vi "update_modifier_values.vi"(0 "TrajectoryDL091126GenericVoxel in":refnum<class "TrajectoryDL091126GenericVoxel.lvclass">, 1 "position-dependently?":bool, 5 "x coordinates in":dbl[unit][](array[numeric]), 7 "y coordinates in":dbl[unit][](array[numeric]), 9 "z coordinates in":dbl[unit][](array[numeric]), 11 "error in (no error)":errorcluster) -> (4 "TrajectoryDL091126GenericVoxel out":refnum<class "TrajectoryDL091126GenericVoxel.lvclass">, 6 "x coordinates out":dbl[unit][](array[numeric]), 8 "y coordindates out":dbl[unit][](array[numeric]), 10 "z coordinates out":dbl[unit][](array[numeric]), 15 "error out":errorcluster)   [LabVIEW 2010, in "TrajectoryDL091126GenericVoxel.lvclass"]
uses:
  TrajectoryDL091126GenericVoxel.lvclass
  common/enumerations/functional_global_action_enum.ctl
  TrajectoryDL091126GenericVoxel.lvclass/TrajectoryDL091126GenericVoxel.ctl
  common/classes/ErrorController/ErrorController/class_data.vi
  common/classes/ErrorController/ErrorController/ErrorController.lvclass
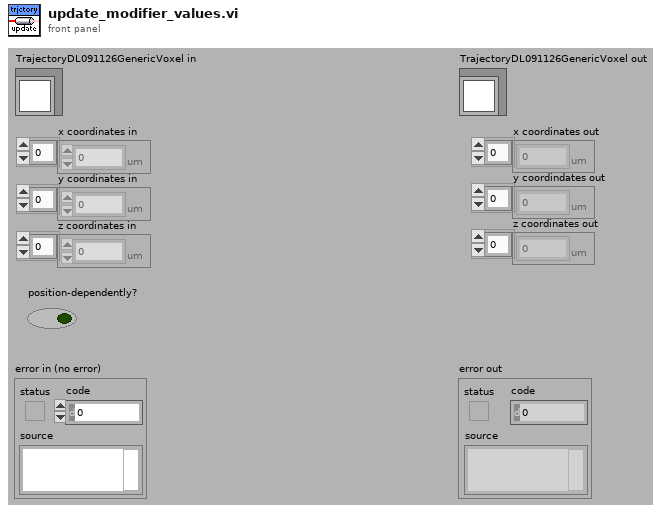
[diagram p1: front panel]
types:
  T1 = typedef "functional_global_action_enum.ctl" = enum16{"get", "set", "reset"}
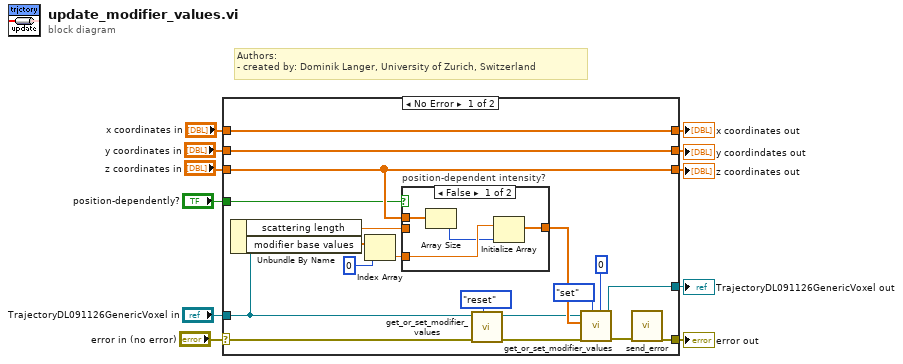
[diagram p0: block diagram]
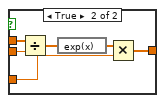
[diagram p2: hidden frame]
diagram:
  # "Authors: \n- created by: Dominik Langer, University of Zurich, Switzerland"
  n1 = case shown="No Error" "error in (no error)" {
    selector: "error in (no error)" -> [w19 w45]
    tunnel: [w13 w45] -> w10
    tunnel: [w23 w44] -> w8
    tunnel: "TrajectoryDL091126GenericVoxel in" -> [w17 w44]
    tunnel: "z coordinates in" -> [w20 w43]
    tunnel: [w20 w43] -> w2
    tunnel: [w22 w41] -> w4
    tunnel: "x coordinates in" -> [w22 w41]
    tunnel: [w21 w42] -> w3
    tunnel: "y coordinates in" -> [w21 w42]
    tunnel: "position-dependently?" -> [w14 _]
    frame No Error {
      n2 = Unbundle By Name(w17) -> ("scattering length"=w24:dbl[unit], "modifier base values"=w25:dbl[])
      n3 = Index Array(array=w25, index=0 ("index (row)")) -> (element=w27:dbl)
      n4 = case "position-dependent intensity?" shown="False" w14 {
        tunnel: [w31 w40] -> w28
        tunnel: w27 -> [w33 w39]
        tunnel: w24 -> [_ w36]
        tunnel: w20 -> [w34 w35]
        frame False {
          n5 = Array Size(array=w34) -> (size(s)=w32:i32)
          n6 = Initialize Array(w33, w32) -> (w31:dbl[])
        }
        frame True {
          n7 = Divide(x=w35, y=w36) -> (x/y=w37:dbl[])
          n8 = expression code="exp(x)"(w37) -> (w38:dbl[])
          n9 = Multiply(x=w38, y=w39) -> (x*y=w40:dbl[])
        }
      }
      n10 = call-dynamic "get_or_set_modifier_values.vi"("action"=functional_global_action_enum."reset", "error in (no error)"=w19, "GenericTrajectory in"=w17) -> ("error out"=w18:errorcluster, "GenericTrajectory out"=w16:refnum<class "TrajectoryDL091126GenericVoxel.lvclass">)  [unwired: 6 in, 1 out]
      n11 = call-dynamic "get_or_set_modifier_values.vi"("modifier index"=0, "action"=functional_global_action_enum."set", "error in (no error)"=w18, "modifier values in"=w28, "GenericTrajectory in"=w16) -> ("error out"=w12:errorcluster, "GenericTrajectory out"=w23:refnum<class "TrajectoryDL091126GenericVoxel.lvclass">)  [unwired: 4 in, 1 out]
      n12 = call "send_error.vi"("error in (no error)"=w12) -> ("error out"=w13:errorcluster)  [unwired: 10 in]
    }
    frame Error {
    }
  }
  "error out" <- w10
  "TrajectoryDL091126GenericVoxel out" <- w8
  "x coordinates out" <- w4
  "y coordindates out" <- w3
  "z coordinates out" <- w2
